vi "GUI - Microscope control.vi"() -> ()   [LabVIEW 2017]
uses:
  <vilib>/DAQmx/write.llb/DAQmx Write (Analog 1D Wfm NChan NSamp).vi
  <vilib>/DAQmx/write.llb/DAQmx Write (Analog 1D DBL NChan 1Samp).vi
  <vilib>/platform/TimedLoop/XDataNode/XDataNode.xnode
  <vilib>/Platform/TimedLoop/XDataNode/nitl_modes.ctl
  <vilib>/Platform/TimedLoop/XDataNode/XDNodeRunTimeDep.lvlib
  <vilib>/Platform/TimedLoop/XDataNode/wakeup.ctl
  <vilib>/Platform/TimedLoop/XDataNode/timing_clust.ctl
  <vilib>/DAQmx/write.llb/DAQmx Write (Digital Bool 1Line 1Point).vi
panel:
  in  "Live":bool
  in  "Snap":bool
  in  "Fast axis frequency":dbl=100.0
  in  "Special coordinates (um)":T1
  in  "Frame Properties":T2={"Height (um)"=50.0, "Width (um)"=50.0, "Y Position (um)"=0.0, "X Position (um)"=0.0, "Y Resolution"=512.0}
  in  "stop Live":bool
  in  "Tab Control":enum32{"Stream", "Z Stack", "T Stack"}(tab)
  in  "stop Stream":bool
  out "Expected time":dbl
  out "Frame rate":dbl
  in  "Number of frames":dbl=1.0
  in  "Acquire Stream":bool
  in  "Starting position (um)":dbl
  in  "Z separation (um)":dbl
  in  "Acquire Stack":bool
  in  "Number of slices":dbl
  out "Frame rate Z":dbl
  out "Expected time Z":dbl
  in  "stop Z stack":bool
  in  "stop T Stack":bool
  in  "Timed acquisition":bool
  out "Expected time 3":dbl
  in  "T separation":dbl=0.1
  in  "Number of frames T Stack":dbl=1.0
  out "Expected separation":dbl
  in  "CLOSE":bool
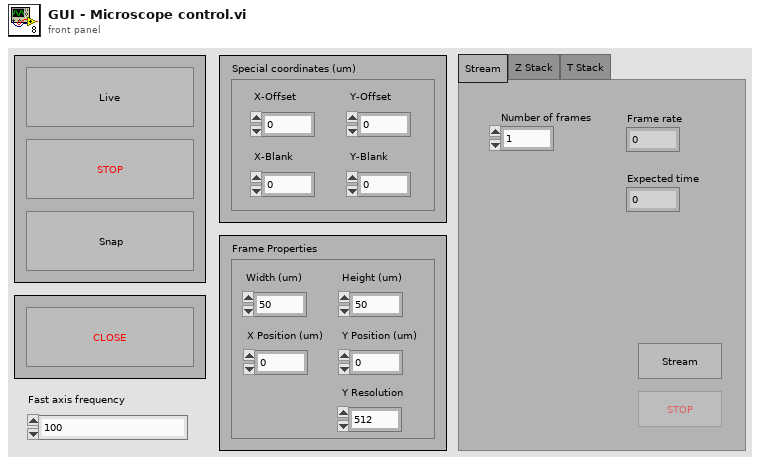
[diagram p1: front panel]
types:
  T1 = cluster{"Y-Offset":dbl, "X-Offset":dbl, "Y-Blank":dbl, "X-Blank":dbl}
  T2 = cluster{"Height (um)":dbl, "Width (um)":dbl, "Y Position (um)":dbl, "X Position (um)":dbl, "Y Resolution":dbl}
  T3 = enum16{"Initialize", "Blank", "Wait for Instructions", "Snap", "Live", "Stream", "T-Stack", "Z-Stack", "Wait for completion", "Stop acquisition", "Close"}
  T4 = enum16{"Wait for instructions", "Blank", "Update parameters", "Update modality", "Scan", "Snap", "Live", "Stream", "T stack", "Z stack", "Close"}
  T5 = enum16{"Wait for instructions", "Blank", "Update parameters", "Update modality", "Scan"}
  T6 = enum16{"Initialize", "Blank", "Wait for Instructions", "Snap", "Live", "T-Stack", "Z-Stack", "Stop acquisition", "Close"}
  T7 = enum16{"Wait for instructions", "Blank", "Update parameters", "Update modality", "Scan", "Close"}
  T8 = typedef "XDNodeRunTimeDep.lvlib/timing_clust.ctl" = cluster{"Expected End [f-1]":u64, "Actual End [f-1]":u64, "Finished Late? [f-1]":bool, "Expected End [i-1]":u64, "Actual End [i-1]":u64, "Finished Late? [i-1]":bool, "Expected Start [i]":u64, "Actual Start [i]":u64, "Expected Start [f]":u64, "Actual Start [f]":u64, "Source Name":string, "Structure Name":string, "Period":i64, "Deadline":i64, "Offset":i64, "Start":i64, "Priority":i32, "Timeout":i32, "Mode":T9, "Wakeup Reason":T10, "Error":errorcluster, "Source Type":string, "Secondary Source Type":string, "Global End Time":u64, "Global Start Time":u64, "Frame Duration":u64, "Iteration Duration":u64, "Assigned CPU":i32, "I/O Scan Engine Mode":u32}
  T9 = typedef "XDNodeRunTimeDep.lvlib/nitl_modes.ctl" = enum32{"No Change", "Process missed periods, maintain original phase", "Discard missed periods, maintain original phase", "Process missed periods, ignore original phase", "Discard missed periods, ignore original phase"}
  T10 = typedef "XDNodeRunTimeDep.lvlib/wakeup.ctl" = enum32{"Normal", "Aborted", "Asynchronous wakeup", "Timing source error", "Timed loop error", "Timeout"}
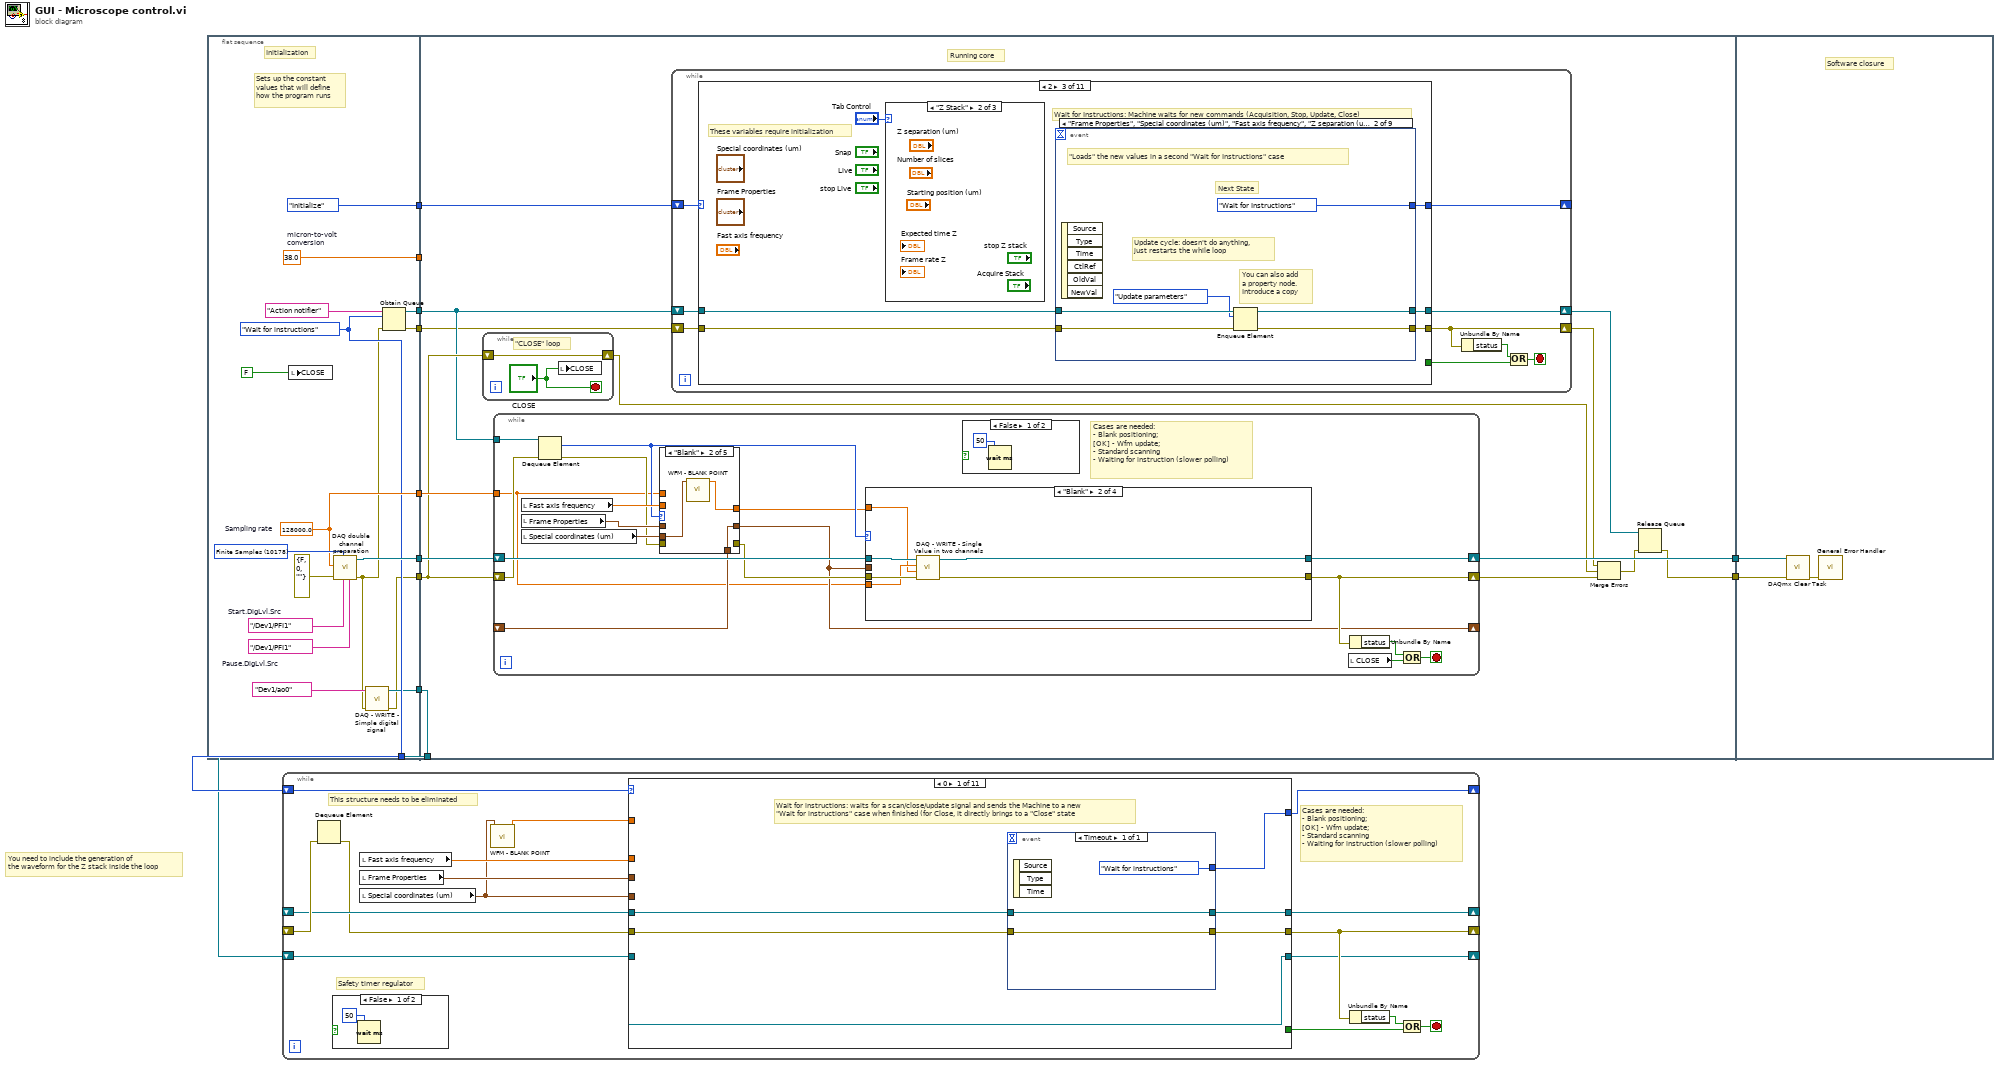
[diagram p0: block diagram]
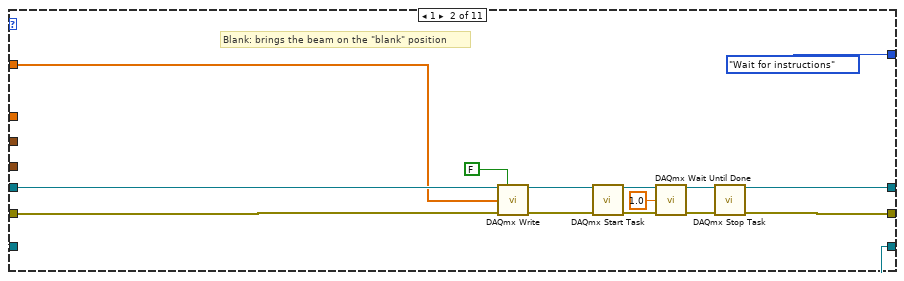
[diagram p2: hidden frame]
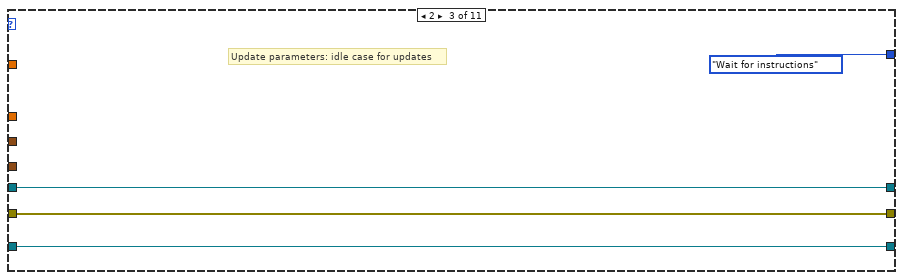
[diagram p3: hidden frame]
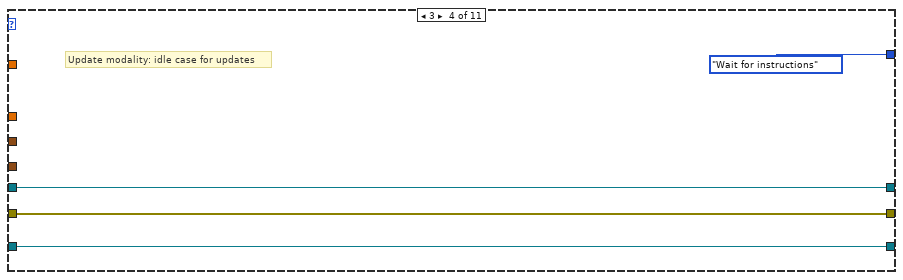
[diagram p4: hidden frame]
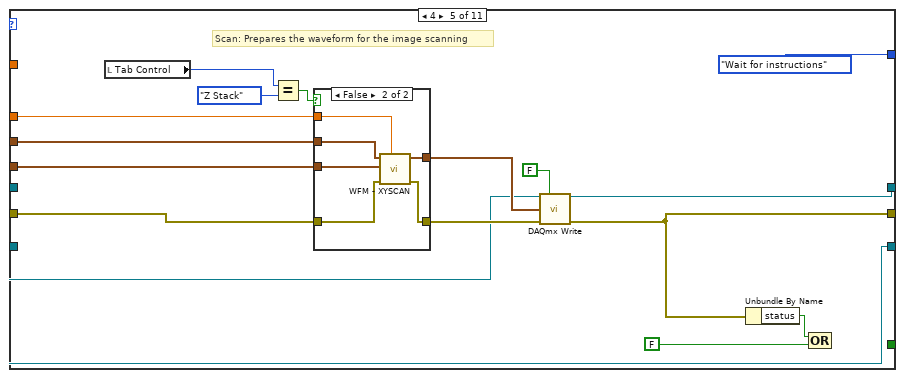
[diagram p5: hidden frame]
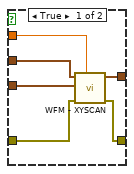
[diagram p6: hidden frame]
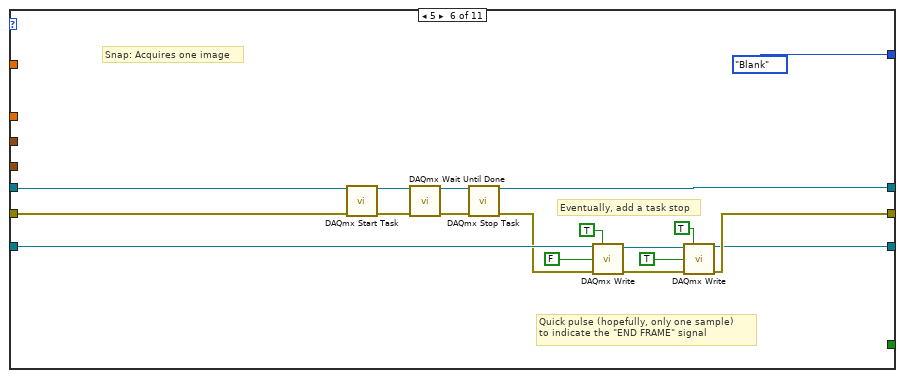
[diagram p7: hidden frame]
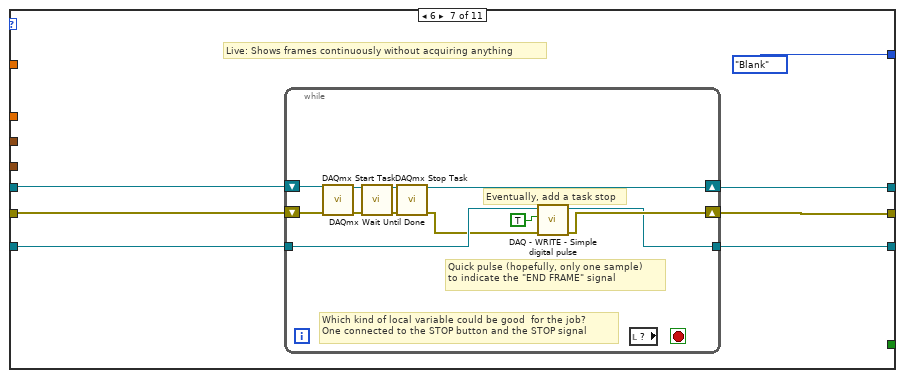
[diagram p8: hidden frame]
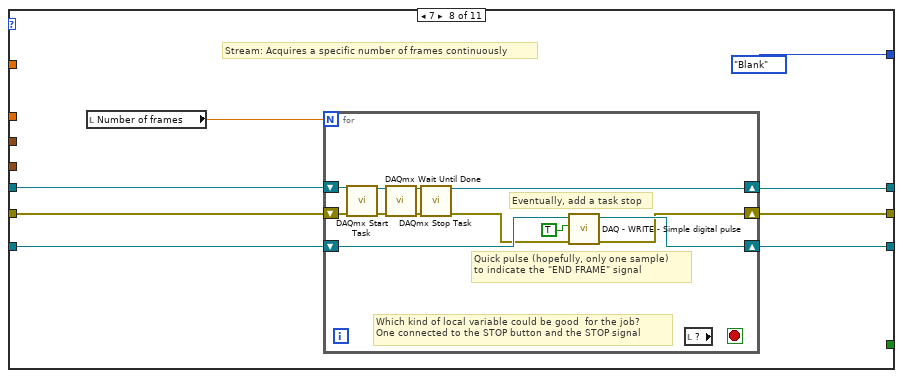
[diagram p9: hidden frame]
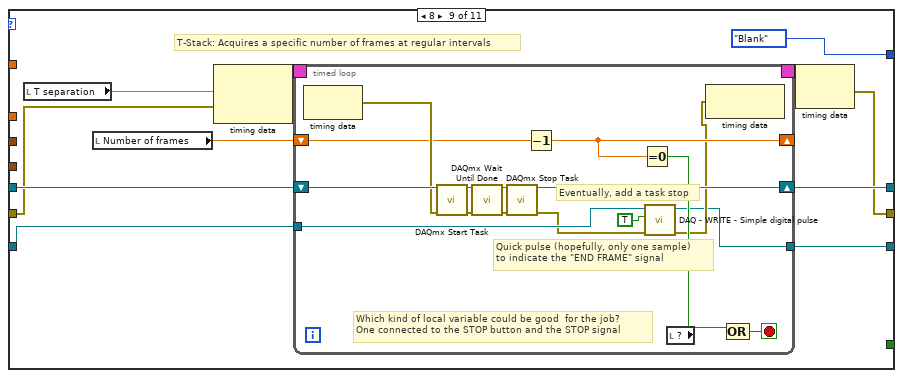
[diagram p10: hidden frame]
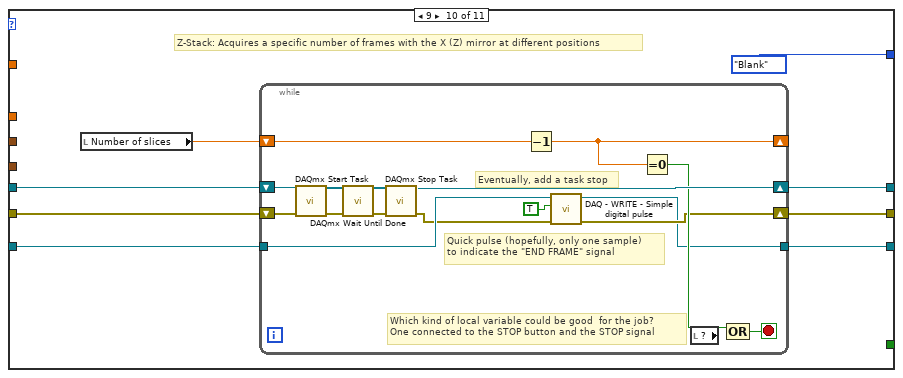
[diagram p11: hidden frame]
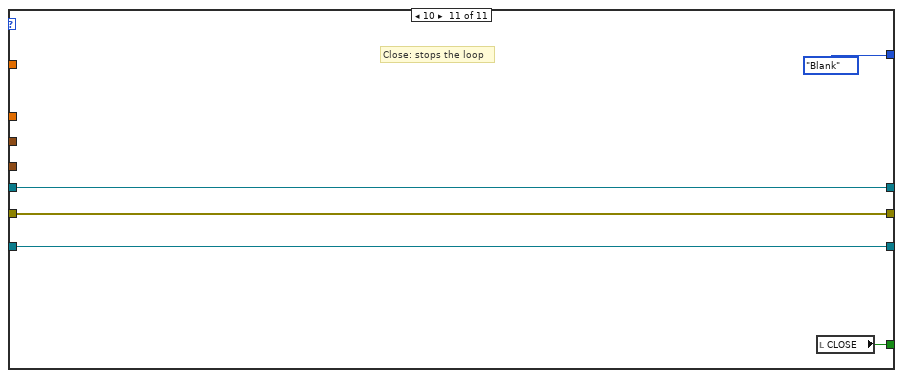
[diagram p12: hidden frame]
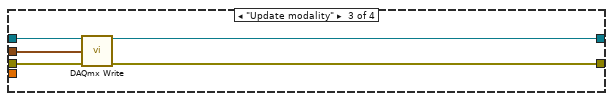
[diagram p15: hidden frame]
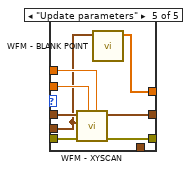
[diagram p20: hidden frame]
diagram:
  # "You need to include the generation of \nthe waveform for the Z stack inside the loop"
  n1 = flat-sequence {
    tunnel: [w27] -> w12
    tunnel: [w13] -> w11
    tunnel: [w25] -> w10
    tunnel: [w24] -> w9
    tunnel: [T3."Initialize"] -> w6
    tunnel: [w20] -> w5
    tunnel: [w19] -> w4
    tunnel: [w17] -> w3
    tunnel: [w15] -> w2
    tunnel: w12 -> [w42]
    tunnel: w11 -> [w36]
    tunnel: w10 -> [w39]
    tunnel: w9 -> [_]
    tunnel: [w33] -> w8
    tunnel: [w41] -> w7
    tunnel: w6 -> [w40]
    tunnel: w5 -> [w32]
    tunnel: w4 -> [w31]
    tunnel: w2 -> [w30]
    tunnel: [w30] -> w1
    tunnel: w8 -> [w222]
    tunnel: w7 -> [w221]
    frame #0 {
      w21 = tag "/Dev1/PFI1"  # Pause.DigLvl.Src
      w17 = T4."Wait for instructions"
      w26 = 10178 items=["Finite Samples"=10178, "Continuous Samples"=10123, "Hardware Timed Single Point"=12522] ("sample mode")
      w22 = tag "/Dev1/PFI1"  # Start.DigLvl.Src
      w24 = 38.0  # micron-to-volt  conversion
      w25 = 128000.0  # Sampling rate
      # "Sets up the constant \nvalues that will define \nhow the program runs"
      # "Initialization"
      n2 = local write "CLOSE"(FALSE) -> ()
      n3 = call "DAQ double channel preparation.vi"("Pause.DigLvl.Src 2"=w21, "Start.DigLvl.Src"=w22, "sample mode"=w26, "error in"=errorcluster {"status"=FALSE, "code"=0, "source"=""}, "rate"=w25) -> ("error out"=w14:errorcluster, "task out"=w27:refnum<k21>)  [unwired: 5 in]
      n4 = call "DAQ - WRITE - Simple digital signal.vi"("error in"=w14, "Digital Output Channel"=tag "Dev1/ao0") -> ("error out"=w13:errorcluster, "task out"=w15:refnum<k21>)  [unwired: 8 in]
      n5 = Obtain Queue(name (unnamed)="Action notifier", element data type=w17, error in (no error)=w14) -> (queue out=w20:refnum<queue>, error out=w19:errorcluster)  [unwired: 2 in, 1 out]
    }
    frame #1 {
      # "Running core"
      n6 = while {
        shift-right: [w44] -> w38
        shift-left: w36 -> [w44]
        stop <- "CLOSE" stop-if-true
        # "\"CLOSE\" loop"
        n7 = local write "CLOSE"("CLOSE") -> ()
      }
      n8 = while {
        shift-right: [w51] -> w43
        shift-left: w36 -> [w56]
        shift-right: [w53] -> w41
        shift-left: w42 -> [w63]
        tunnel: w39 -> [w47]
        shift-right: [w50] -> _
        shift-left: _ -> [w54]
        tunnel: w32 -> [w48]
        stop <- w61 stop-if-true
        # "Cases are needed: \n- Blank positioning; \n[OK] - Wfm update; \n- Standard scanning\n- Waiting for instruction (slower polling)"
        n9 = local read "Fast axis frequency"() -> (w59:dbl)
        n10 = local read "Frame Properties"() -> (w57:T2)
        n11 = local read "Special coordinates (um)"() -> (w58:T1)
        n12 = Dequeue Element(queue=w48, error in (no error)=w56) -> (element=w49:T4, error out=w55:errorcluster)  [unwired: 1 in, 2 out]
        n13 = case shown="\"Blank\"" w49 {
          tunnel: [_ _ _ _ w90] -> w52
          tunnel: w59 -> [_ _ _ _ w89]
          tunnel: w58 -> [_ w79 _ _ w84]
          tunnel: w57 -> [_ _ _ _ w87]
          tunnel: [w77 w80 w81 w82 w88] -> w50
          tunnel: w47 -> [_ _ _ _ w86]
          tunnel: w55 -> [_ _ _ _ w85]
          tunnel: w54 -> [w77 w80 w81 w82 _]
          tunnel: [_ w78 _ _ w83] -> w46
          frame "Wait for instructions", Default {
          }
          frame "Blank" {
            n14 = call "WFM - BLANK POINT.vi"("Special coordinates (um)"=w79) -> ("appended array"=w78:dbl[])  [unwired: 10 in]
          }
          frame "Update modality" {
          }
          frame "Scan" {
          }
          frame "Update parameters" {
            n15 = call "WFM - XYSCAN.vi"("Sampling rate"=w86, "Fast axis frequency"=w89, "error in (no error)"=w85, "Special coordinates (um)"=w84, "Frame Properties"=w87) -> ("error out"=w90:errorcluster, "appended array"=w88:waveform(dbl)[])  [unwired: 5 in]
            n16 = call "WFM - BLANK POINT.vi"("Special coordinates (um)"=w84) -> ("appended array"=w83:dbl[])  [unwired: 10 in]
          }
        }
        n17 = case shown="\"Blank\"" w49 {
          tunnel: w63 -> [w65 w71 w76 _]
          tunnel: [w65 w69 w75 _] -> w53
          tunnel: w52 -> [w64 w70 w74 _]
          tunnel: [w64 w68 w73 _] -> w51
          tunnel: w50 -> [_ _ w72 _]
          tunnel: w47 -> [_ w67 _ _]
          tunnel: w46 -> [_ w66 _ _]
          frame "Wait for instructions", Default {
          }
          frame "Blank" {
            n18 = call "DAQ - WRITE - Single Value in two channels.vi"("error in"=w70, "data"=w66, "rate"=w67, "task/channels in"=w71) -> ("error out"=w68:errorcluster, "task out"=w69:refnum<k21>)  [unwired: 6 in]
          }
          frame "Update modality" {
            n19 = call-poly <vilib>:"DAQmx Write.vi"("task/channels in"=w76, "data"=w72, "error in"=w74) -> ("task out"=w75:refnum<k21>, "error out"=w73:errorcluster)  [unwired: 10 in, 1 out]
          }
          frame "Scan" {
          }
        }
        n20 = case shown="False" {
          selector: _ -> [_ _]
          frame False {
            n21 = Wait (ms)(milliseconds to wait=50) -> ()  [unwired: 1 out]
          }
          frame True {
            # "Acquisition (Consumer)"
          }
        }
        n22 = local read "CLOSE"() -> (w62:bool)
        n23 = Unbundle By Name(w51) -> ("status"=w60:bool)
        n24 = Compound Arithmetic op=OR(w60, w62) -> (w61:bool)
      }
      n25 = while {
        shift-right: [w97] -> w37
        shift-left: w31 -> [w100]
        shift-right: [w95] -> _
        shift-left: w40 -> [w92]
        shift-right: [w93] -> w35
        shift-left: w32 -> [w94]
        stop <- w99 stop-if-true
        n26 = case shown="2" w92 {
          tunnel: w100 -> [w103 w105 w110 w173 w180 w185 w192 w199 w201 w211 w218]
          tunnel: [w103 w106 w115 w172 w179 w184 w191 w198 w202 w210 w215] -> w97
          tunnel: [_ _ _ _ _ _ _ _ _ _ w220] -> w96
          tunnel: [T3."Blank" T3."Wait for Instructions" w114 T3."Wait for completion" T3."Wait for completion" T3."Wait for completion" T3."Wait for completion" T3."Wait for completion" w206 T3."Blank" T6."Initialize"] -> w95
          tunnel: w94 -> [w102 w108 w112 w175 w182 w187 w193 w200 w204 w212 w217]
          tunnel: [w102 w107 w111 w174 w181 w186 w190 w197 w203 w209 w216] -> w93
          frame 0 {
            (unwired) T4."Wait for instructions"
            # "Initialize phase: sends the Machine to the \"Blank\" state"
            # "Next State"
          }
          frame 1 {
            # "Blank phase: brings the beam on the blank position and sends the Machine to \"Wait for Instructions\""
            # "Next State"
            n27 = Enqueue Element(queue=w108, element=T4."Blank", error in (no error)=w105) -> (queue out=w107:refnum<queue>, error out=w106:errorcluster)  [unwired: 1 in, 1 out]
          }
          frame 2 {
            # "Wait for Instructions: Machine waits for new commands (Acquisition, Stop, Update, Close)"
            # "These variables require initialization"
            n28 = case shown="\"Z Stack\"" "Tab Control" {
              frame "Stream" {
                n29 = Multiply(x="Number of frames") -> (x*y=→"Expected time":dbl)  [unwired: 1 in]
              }
              frame "Z Stack" {
              }
              frame "T Stack" {
                n30 = Multiply(x="Number of frames T Stack") -> (x*y=→"Expected separation":dbl)  [unwired: 1 in]
              }
            }
            n31 = event shown="[1] \"Frame Properties\", \"Special coordinates (um)\", \"Fast axis frequency\", \"Z separation (um)\", \"Number of slices\", \"Starting position (um)\": Value Change" {
              selector: _ -> [_ _ _ _ _ _ _ _ _]
              dyn-events: _ -> [_ _ _ _ _ _ _ _ _]
              timeout: _ -> [_ _ _ _ _ _ _ _ _]
              tunnel: w110 -> [w122 w128 w132 w138 w144 w150 w156 w162 w168]
              tunnel: [w122 w127 w130 w136 w142 w148 w154 w160 w166] -> w115
              tunnel: [T3."Close" T3."Wait for Instructions" T3."Wait for Instructions" T3."Snap" T3."Live" T3."Stream" T3."T-Stack" T3."Z-Stack" T3."Wait for Instructions"] -> w114
              tunnel: w112 -> [w121 w126 w133 w139 w145 w151 w157 w163 w169]
              tunnel: [w121 w125 w131 w137 w143 w149 w155 w161 w167] -> w111
              event "CLOSE": Value Change {
                # "Brings the Machine to the \"Close\" state"
                # "Next State"
                n32 = event-data() -> ()  [unwired: 1 in, 5 out]
              }
              event "Frame Properties", "Special coordinates (um)", "Fast axis frequency", "Z separation (um)", "Number of slices", "Starting position (um)": Value Change {
                # "\"Loads\" the new values in a second \"Wait for Instructions\" case"
                # "You can also add \na property node. \nIntroduce a copy"
                # "Next State"
                # "Update cycle: doesn't do anything, \njust restarts the while loop"
                n33 = event-data() -> ()  [unwired: 1 in, 6 out]
                n34 = Enqueue Element(queue=w126, element=T5."Update parameters" ("kkk;lkl;"), error in (no error)=w128) -> (queue out=w125:refnum<queue>, error out=w127:errorcluster)  [unwired: 1 in, 1 out]
              }
              event "Tab Control", "T separation", "Number of frames T Stack", "Z separation (um)", "Number of slices", "Number of frames": Value Change {
                # "\"Loads\" the new modality in a second \"Wait for Instructions\" case"
                # "Next State"
                # "Update cycle: doesn't do anything, \njust restarts the while loop"
                n35 = event-data() -> ()  [unwired: 1 in, 6 out]
                n36 = Enqueue Element(queue=w133, element=T5."Update modality" ("kkk;lkl;"), error in (no error)=w132) -> (queue out=w131:refnum<queue>, error out=w130:errorcluster)  [unwired: 1 in, 1 out]
              }
              event "Snap": Value Change {
                # "Gives the command for a snapshot and brings the Machine to the \"Wait for completion\" state"
                # "Next State"
                n37 = event-data() -> ()  [unwired: 1 in, 6 out]
                n38 = Enqueue Element(queue=w139, element=T5."Scan" ("kkk;lkl;"), error in (no error)=w138) -> (queue out=w137:refnum<queue>, error out=w136:errorcluster)  [unwired: 1 in, 1 out]
              }
              event "Live": Value Change {
                # "Gives the command for a continuous observation (without acquisition) and brings the Machine to the \"Wait for completion\" state"
                # "Next State"
                n39 = event-data() -> ()  [unwired: 1 in, 6 out]
                n40 = Enqueue Element(queue=w145, element=T5."Scan" ("kkk;lkl;"), error in (no error)=w144) -> (queue out=w143:refnum<queue>, error out=w142:errorcluster)  [unwired: 1 in, 1 out]
              }
              event "Acquire Stream": Value Change {
                # "Gives the command for a continuous observation and acquisition and brings the Machine to the \"Wait for completion\" state"
                # "Next State"
                n41 = event-data() -> ()  [unwired: 1 in, 6 out]
                n42 = Enqueue Element(queue=w151, element=T5."Scan" ("kkk;lkl;"), error in (no error)=w150) -> (queue out=w149:refnum<queue>, error out=w148:errorcluster)  [unwired: 1 in, 1 out]
              }
              event "Timed acquisition": Value Change {
                # "Gives the command for a Timed acquisition and brings the Machine to the \"Wait for completion\" state"
                # "Next State"
                n43 = event-data() -> ()  [unwired: 1 in, 6 out]
                n44 = Enqueue Element(queue=w157, element=T5."Scan" ("kkk;lkl;"), error in (no error)=w156) -> (queue out=w155:refnum<queue>, error out=w154:errorcluster)  [unwired: 1 in, 1 out]
              }
              event "Acquire Stack": Value Change {
                # "Gives the command for a vertical acquisition and brings the Machine to the \"Wait for completion\" state"
                # "Next State"
                n45 = event-data() -> ()  [unwired: 1 in, 6 out]
                n46 = Enqueue Element(queue=w163, element=T5."Scan" ("kkk;lkl;"), error in (no error)=w162) -> (queue out=w161:refnum<queue>, error out=w160:errorcluster)  [unwired: 1 in, 1 out]
              }
              event "stop Live", "stop Stream", "stop T Stack", "stop Z stack": Value Change {
                # "Dummy Case to avoid effects from pressing the STOP buttons  during the idle phase"
                # "Next State"
                n47 = event-data() -> ()  [unwired: 1 in, 6 out]
                n48 = Enqueue Element(queue=w169, element=T5."Wait for instructions" ("kkk;lkl;"), error in (no error)=w168) -> (queue out=w167:refnum<queue>, error out=w166:errorcluster)  [unwired: 1 in, 1 out]
              }
            }
          }
          frame 3 {
            # "Snap: sends the command to take a snapshot and sends the Machine to wait for completion mode"
            # "Next State"
            n49 = Enqueue Element(queue=w175, element=T4."Snap", error in (no error)=w173) -> (queue out=w174:refnum<queue>, error out=w172:errorcluster)  [unwired: 1 in, 1 out]
          }
          frame 4 {
            # "Live: sends the command to start a continuous observation (without acquisition) and sends the Machine to wait for completion mode"
            # "Next State"
            n50 = Enqueue Element(queue=w182, element=T4."Live", error in (no error)=w180) -> (queue out=w181:refnum<queue>, error out=w179:errorcluster)  [unwired: 1 in, 1 out]
          }
          frame 5 {
            # "Stream: sends the command to take a continuous acquisition and sends the Machine to wait for completion mode"
            # "Next State"
            n51 = Enqueue Element(queue=w187, element=T4."Stream", error in (no error)=w185) -> (queue out=w186:refnum<queue>, error out=w184:errorcluster)  [unwired: 1 in, 1 out]
          }
          frame 6 {
            # "T Stack: sends the command to take a timed acquisition and sends the Machine to wait for completion mode"
            # "Next State"
            n52 = Enqueue Element(queue=w193, element=T4."T stack", error in (no error)=w192) -> (queue out=w190:refnum<queue>, error out=w191:errorcluster)  [unwired: 1 in, 1 out]
          }
          frame 7 {
            # "Z Stack: sends the command to take a vertical acquisition and sends the Machine to wait for completion mode"
            # "Next State"
            n53 = Enqueue Element(queue=w200, element=T4."Z stack", error in (no error)=w199) -> (queue out=w197:refnum<queue>, error out=w198:errorcluster)  [unwired: 1 in, 1 out]
          }
          frame 8 {
            # "NEED TO ADD THE END SIGNAL CASE!!!!\nIt needs to go to the state 2, \"Blank\""
            # "Wait for Completion: waits for an \"Acquisition END\" or a \"STOP\" signal and sends the Machine to the \"Wait for instructions\" mode"
            n54 = Enqueue Element(queue=w204, element=T5."Wait for instructions" ("kkk;lkl;"), error in (no error)=w201) -> (queue out=w203:refnum<queue>, error out=w202:errorcluster)  [unwired: 1 in, 1 out]
            n55 = event shown="[1] \"CLOSE\": Value Change" {
              selector: _ -> [_ _]
              dyn-events: _ -> [_ _]
              timeout: _ -> [_ _]
              tunnel: [T3."Stop acquisition" T3."Close"] -> w206
              event "stop T Stack", "stop Z stack", "stop Stream", "stop Live": Value Change {
                # "Next State"
                n56 = event-data() -> ()  [unwired: 1 in, 6 out]
              }
              event "CLOSE": Value Change {
                # "Next State"
                n57 = event-data() -> ()  [unwired: 1 in, 6 out]
              }
            }
          }
          frame 9 {
            # "Stop Acquisition: generates a \"stop acquisition signal\" and sends the Machine to wait for completion mode"
            # "Next State"
            n58 = Enqueue Element(queue=w212, element=T5."Wait for instructions" ("kkk;lkl;"), error in (no error)=w211) -> (queue out=w209:refnum<queue>, error out=w210:errorcluster)  [unwired: 1 in, 1 out]
          }
          frame 10 {
            (unwired) T7."Close"
            # "Close: stops the software"
            # "Next State (It won't be read)"
            n59 = Enqueue Element(queue=w217, error in (no error)=w218) -> (queue out=w216:refnum<queue>, error out=w215:errorcluster)  [unwired: 2 in, 1 out]
            n60 = local read "CLOSE"() -> (w220:bool)
          }
        }
        n61 = Unbundle By Name(w97) -> ("status"=w98:bool)
        n62 = Compound Arithmetic op=OR(w98, w96) -> (w99:bool)
      }
      n63 = Merge Errors(w37, w38, w43) -> (w34:errorcluster)
      n64 = Release Queue(queue=w35, error in (no error)=w34) -> (error out=w33:errorcluster)  [unwired: 1 in, 2 out]
    }
    frame #2 {
      # "Software closure"
      n65 = call <vilib>:"DAQmx Clear Task.vi"("task in"=w221, "error in"=w222) -> ("error out"=w223:errorcluster)  [unwired: 13 in]
      n66 = call <vilib>:"General Error Handler.vi"("error in (no error)"=w223) -> ()  [unwired: 10 in, 5 out]
    }
  }
  n67 = while {
    shift-right: [w236] -> _
    shift-left: _ -> [w237]
    shift-right: [w234] -> _
    shift-left: _ -> [w235]
    shift-right: [w232] -> _
    shift-left: w3 -> [w228]
    shift-right: [w224] -> _
    shift-left: w1 -> [w225]
    stop <- w239 stop-if-true
    # "Safety timer regulator"
    # "This structure needs to be eliminated"
    # "Cases are needed: \n- Blank positioning; \n[OK] - Wfm update; \n- Standard scanning\n- Waiting for instruction (slower polling)"
    n68 = Dequeue Element(error in (no error)=w237) -> (error out=w227:errorcluster)  [unwired: 2 in, 3 out]
    n69 = case shown="False" {
      selector: _ -> [_ _]
      frame False {
        n70 = Wait (ms)(milliseconds to wait=50) -> ()  [unwired: 1 out]
      }
      frame True {
        # "Acquisition (Consumer)"
      }
    }
    n71 = local read "Fast axis frequency"() -> (w231:dbl)
    n72 = local read "Frame Properties"() -> (w230:T2)
    n73 = local read "Special coordinates (um)"() -> (w229:T1)
    n74 = call "WFM - BLANK POINT.vi"("Special coordinates (um)"=w229) -> ("appended array"=w226:dbl[])  [unwired: 10 in]
    n75 = case shown="0" w228 {
      tunnel: w227 -> [w245 w262 w267 w271 w278 w313 w324 w344 w363 w399 w424]
      tunnel: [w244 w254 w267 w271 w287 w303 w321 w341 w362 w398 w424] -> w236
      tunnel: [w243 w258 w266 w270 w288 w311 w322 w342 w366 w401 w423] -> w234
      tunnel: w235 -> [w242 w263 w266 w270 w276 w312 w323 w343 w367 w402 w423]
      tunnel: [_ _ _ _ _ _ _ _ _ _ w422] -> w233
      tunnel: [w241 T7."Wait for instructions" T4."Wait for instructions" T4."Wait for instructions" T4."Wait for instructions" T4."Blank" T4."Blank" T4."Blank" T4."Blank" T4."Blank" T7."Blank"] -> w232
      tunnel: w231 -> [_ _ _ _ w283 _ _ _ _ _ _]
      tunnel: w229 -> [_ _ _ _ w282 _ _ _ _ _ _]
      tunnel: w230 -> [_ _ _ _ w281 _ _ _ _ _ _]
      tunnel: w226 -> [_ w250 _ _ _ _ _ _ _ _ _]
      tunnel: w225 -> [w240 w249 w264 w268 w272 w310 w320 w339 w359 w397 w420]
      tunnel: [w240 w249 w264 w268 w272 w301 w319 w338 w358 w396 w420] -> w224
      frame 0 {
        # "Wait for instructions: waits for a scan/close/update signal and sends the Machine to a new \n\"Wait for instructions\" case when finished (for Close, it directly brings to a \"Close\" state"
        n76 = event shown="[0] Timeout" {
          selector: _ -> [_]
          dyn-events: _ -> [_]
          timeout: _ -> [_]
          tunnel: w245 -> [w248]
          tunnel: [w248] -> w244
          tunnel: w242 -> [w247]
          tunnel: [w247] -> w243
          tunnel: [T7."Wait for instructions"] -> w241
          event Timeout {
            n77 = event-data() -> ()  [unwired: 1 in, 3 out]
          }
        }
      }
      frame 1 {
        # "Blank: brings the beam on the \"blank\" position"
        n78 = call-poly <vilib>:"DAQmx Write.vi"("task/channels in"=w263, "auto start"=FALSE, "data"=w250, "error in"=w262) -> ("task out"=w261:refnum<k21>, "error out"=w257:errorcluster)  [unwired: 9 in, 1 out]
        n79 = call <vilib>:"DAQmx Start Task.vi"("task/channels in"=w261, "error in"=w257) -> ("task out"=w260:refnum<k21>, "error out"=w256:errorcluster)  [unwired: 12 in]
        n80 = call <vilib>:"DAQmx Wait Until Done.vi"("task/channels in"=w260, "timeout (sec)"=1.0, "error in"=w256) -> ("task out"=w259:refnum<k21>, "error out"=w255:errorcluster)  [unwired: 11 in]
        n81 = call <vilib>:"DAQmx Stop Task.vi"("task/channels in"=w259, "error in"=w255) -> ("task out"=w258:refnum<k21>, "error out"=w254:errorcluster)  [unwired: 12 in]
      }
      frame 2 {
        # "Update parameters: idle case for updates"
      }
      frame 3 {
        # "Update modality: idle case for updates"
      }
      frame 4 {
        # "Scan: Prepares the waveform for the image scanning"
        n82 = local read "Tab Control"() -> (w275:enum32{"Stream", "Z Stack", "T Stack"})
        n83 = Equal?(x=w275, y=enum32{"Stream", "Z Stack", "T Stack"}."Z Stack") -> (x = y?=w273:bool)
        n84 = case shown="False" w273 {
          tunnel: w283 -> [w294 w300]
          tunnel: w282 -> [w293 w299]
          tunnel: w281 -> [w292 w298]
          tunnel: [w291 w297] -> w280
          tunnel: [w290 w296] -> w279
          tunnel: w278 -> [w289 w295]
          frame True {
            n85 = call "WFM - XYSCAN.vi"("Fast axis frequency"=w294, "error in (no error)"=w289, "Special coordinates (um)"=w293, "Frame Properties"=w292) -> ("error out"=w291:errorcluster, "appended array"=w290:waveform(dbl)[])  [unwired: 6 in]
          }
          frame False {
            n86 = call "WFM - XYSCAN.vi"("Fast axis frequency"=w300, "error in (no error)"=w295, "Special coordinates (um)"=w299, "Frame Properties"=w298) -> ("error out"=w297:errorcluster, "appended array"=w296:waveform(dbl)[])  [unwired: 6 in]
          }
        }
        n87 = call-poly <vilib>:"DAQmx Write.vi"("task/channels in"=w276, "auto start"=FALSE, "data"=w279, "error in"=w280) -> ("task out"=w288:refnum<k21>, "error out"=w287:errorcluster)  [unwired: 9 in, 1 out]
        n88 = Unbundle By Name(w287) -> ("status"=w284:bool)
        n89 = Compound Arithmetic op=OR(w284, FALSE) -> ()  [unwired: 1 out]
      }
      frame 5 {
        # "Eventually, add a task stop"
        # "Quick pulse (hopefully, only one sample)\nto indicate the \"END FRAME\" signal"
        # "Snap: Acquires one image"
        n90 = call <vilib>:"DAQmx Start Task.vi"("task/channels in"=w312, "error in"=w313) -> ("task out"=w314:refnum<k21>, "error out"=w316:errorcluster)  [unwired: 12 in]
        n91 = call <vilib>:"DAQmx Wait Until Done.vi"("task/channels in"=w314, "error in"=w316) -> ("task out"=w315:refnum<k21>, "error out"=w317:errorcluster)  [unwired: 12 in]
        n92 = call <vilib>:"DAQmx Stop Task.vi"("task/channels in"=w315, "error in"=w317) -> ("task out"=w311:refnum<k21>, "error out"=w309:errorcluster)  [unwired: 12 in]
        n93 = call-poly <vilib>:"DAQmx Write.vi"("task/channels in"=w310, "auto start"=TRUE, "data"=FALSE, "error in"=w309) -> ("task out"=w302:refnum<k21>, "error out"=w304:errorcluster)  [unwired: 9 in, 1 out]
        n94 = call-poly <vilib>:"DAQmx Write.vi"("task/channels in"=w302, "auto start"=TRUE, "data"=TRUE, "error in"=w304) -> ("task out"=w301:refnum<k21>, "error out"=w303:errorcluster)  [unwired: 9 in, 1 out]
      }
      frame 6 {
        # "Live: Shows frames continuously without acquiring anything"
        n95 = while {
          shift-right: [w327] -> w321
          shift-left: w324 -> [w333]
          shift-right: [w331] -> w322
          shift-left: w323 -> [w332]
          tunnel: w320 -> [w329]
          tunnel: [w326] -> w319
          stop <- _ stop-if-true
          # "Eventually, add a task stop"
          # "Quick pulse (hopefully, only one sample)\nto indicate the \"END FRAME\" signal"
          # "Which kind of local variable could be good  for the job?\nOne connected to the STOP button and the STOP signal"
          n96 = call <vilib>:"DAQmx Start Task.vi"("task/channels in"=w332, "error in"=w333) -> ("task out"=w334:refnum<k21>, "error out"=w336:errorcluster)  [unwired: 12 in]
          n97 = call <vilib>:"DAQmx Wait Until Done.vi"("task/channels in"=w334, "error in"=w336) -> ("task out"=w335:refnum<k21>, "error out"=w337:errorcluster)  [unwired: 12 in]
          n98 = call <vilib>:"DAQmx Stop Task.vi"("task/channels in"=w335, "error in"=w337) -> ("task out"=w331:refnum<k21>, "error out"=w328:errorcluster)  [unwired: 12 in]
          n99 = call "DAQ - WRITE - Simple digital pulse.vi"("error in"=w328, "data"=TRUE, "task/channels in"=w329) -> ("error out"=w327:errorcluster, "task out"=w326:refnum<k21>)  [unwired: 7 in]
          n100 = local read item#-1() -> ()  [unwired: 1 out]
        }
      }
      frame 7 {
        # "Stream: Acquires a specific number of frames continuously"
        n101 = local read "Number of frames"() -> (w340:dbl)
        n102 = for {
          N: w340 -> [_]
          shift-right: [w346] -> w341
          shift-left: w344 -> [w353]
          shift-right: [w351] -> w342
          shift-left: w343 -> [w352]
          shift-right: [w347] -> w338
          shift-left: w339 -> [w349]
          stop <- _ stop-if-true
          # "Eventually, add a task stop"
          # "Quick pulse (hopefully, only one sample)\nto indicate the \"END FRAME\" signal"
          # "Which kind of local variable could be good  for the job?\nOne connected to the STOP button and the STOP signal"
          n103 = call <vilib>:"DAQmx Start Task.vi"("task/channels in"=w352, "error in"=w353) -> ("task out"=w354:refnum<k21>, "error out"=w356:errorcluster)  [unwired: 12 in]
          n104 = call <vilib>:"DAQmx Wait Until Done.vi"("task/channels in"=w354, "error in"=w356) -> ("task out"=w355:refnum<k21>, "error out"=w357:errorcluster)  [unwired: 12 in]
          n105 = call <vilib>:"DAQmx Stop Task.vi"("task/channels in"=w355, "error in"=w357) -> ("task out"=w351:refnum<k21>, "error out"=w348:errorcluster)  [unwired: 12 in]
          n106 = call "DAQ - WRITE - Simple digital pulse.vi"("error in"=w348, "data"=TRUE, "task/channels in"=w349) -> ("error out"=w346:errorcluster, "task out"=w347:refnum<k21>)  [unwired: 7 in]
          n107 = local read item#-1() -> ()  [unwired: 1 out]
        }
      }
      frame 8 {
        # "T-Stack: Acquires a specific number of frames at regular intervals"
        n108 = local read "T separation"() -> (w361:dbl)
        n109 = local read "Number of frames"() -> (w360:dbl)
        n110 = node-c288(w361, w363) -> (w365:T8)
        n111 = timed-loop {
          timing: w365 -> [_]
          timing-out: [_] -> w364
          shift-right: [w375] -> _
          shift-left: w360 -> [w377]
          shift-right: [w383] -> w366
          shift-left: w367 -> [w384]
          tunnel: w359 -> [w372]
          tunnel: [w369] -> w358
          stop <- w376 stop-if-true
          # "Eventually, add a task stop"
          # "Quick pulse (hopefully, only one sample)\nto indicate the \"END FRAME\" signal"
          # "Which kind of local variable could be good  for the job?\nOne connected to the STOP button and the STOP signal"
          n112 = node-c288() -> (w378:errorcluster)  [unwired: 1 in]
          n113 = call <vilib>:"DAQmx Start Task.vi"("task/channels in"=w384, "error in"=w378) -> ("task out"=w379:refnum<k21>, "error out"=w381:errorcluster)  [unwired: 12 in]
          n114 = call <vilib>:"DAQmx Wait Until Done.vi"("task/channels in"=w379, "error in"=w381) -> ("task out"=w380:refnum<k21>, "error out"=w382:errorcluster)  [unwired: 12 in]
          n115 = call <vilib>:"DAQmx Stop Task.vi"("task/channels in"=w380, "error in"=w382) -> ("task out"=w383:refnum<k21>, "error out"=w371:errorcluster)  [unwired: 12 in]
          n116 = Decrement(x=w377) -> (x-1=w375:dbl)
          n117 = Equal To 0?(x=w375) -> (x = 0?=w374:bool)
          n118 = call "DAQ - WRITE - Simple digital pulse.vi"("error in"=w371, "data"=TRUE, "task/channels in"=w372) -> ("error out"=w370:errorcluster, "task out"=w369:refnum<k21>)  [unwired: 7 in]
          n119 = local read item#-1() -> ()  [unwired: 1 out]
          n120 = node-c288(w370) -> ()  [unwired: 1 out]
          n121 = Compound Arithmetic op=OR(w374) -> (w376:bool)  [unwired: 1 in]
        }
        n122 = node-c288(w364) -> (w362:errorcluster)
      }
      frame 9 {
        # "Z-Stack: Acquires a specific number of frames with the X (Z) mirror at different positions"
        n123 = local read "Number of slices"() -> (w400:dbl)
        n124 = while {
          shift-right: [w411] -> _
          shift-left: w400 -> [w413]
          shift-right: [w405] -> w398
          shift-left: w399 -> [w409]
          shift-right: [w418] -> w401
          shift-left: w402 -> [w419]
          tunnel: w397 -> [w407]
          tunnel: [w404] -> w396
          stop <- w412 stop-if-true
          # "Eventually, add a task stop"
          # "Quick pulse (hopefully, only one sample)\nto indicate the \"END FRAME\" signal"
          # "Which kind of local variable could be good  for the job?\nOne connected to the STOP button and the STOP signal"
          n125 = call <vilib>:"DAQmx Start Task.vi"("task/channels in"=w419, "error in"=w409) -> ("task out"=w414:refnum<k21>, "error out"=w416:errorcluster)  [unwired: 12 in]
          n126 = call <vilib>:"DAQmx Wait Until Done.vi"("task/channels in"=w414, "error in"=w416) -> ("task out"=w415:refnum<k21>, "error out"=w417:errorcluster)  [unwired: 12 in]
          n127 = call <vilib>:"DAQmx Stop Task.vi"("task/channels in"=w415, "error in"=w417) -> ("task out"=w418:refnum<k21>, "error out"=w406:errorcluster)  [unwired: 12 in]
          n128 = Decrement(x=w413) -> (x-1=w411:dbl)
          n129 = call "DAQ - WRITE - Simple digital pulse.vi"("error in"=w406, "data"=TRUE, "task/channels in"=w407) -> ("error out"=w405:errorcluster, "task out"=w404:refnum<k21>)  [unwired: 7 in]
          n130 = Equal To 0?(x=w411) -> (x = 0?=w410:bool)
          n131 = local read item#-1() -> ()  [unwired: 1 out]
          n132 = Compound Arithmetic op=OR(w410) -> (w412:bool)  [unwired: 1 in]
        }
      }
      frame 10 {
        # "Close: stops the loop"
        n133 = local read "CLOSE"() -> (w422:bool)
      }
    }
    n134 = Unbundle By Name(w236) -> ("status"=w238:bool)
    n135 = Compound Arithmetic op=OR(w238, w233) -> (w239:bool)
  }
